vi "send_scan_data_to_AnalysisObj.vi"(0 "SessionID":string, 5 "plotname":string, 7 "magnet value in":dbl, 9 "value":dbl, 11 "error in (no error)":errorcluster) -> (15 "error out":errorcluster)   [LabVIEW 2017]
doc: "sendds the data to the AnalysisSession (SessionID) and stores them in the ScanDataArray"
uses:
  Classes/Analysis/Analysis.lvclass
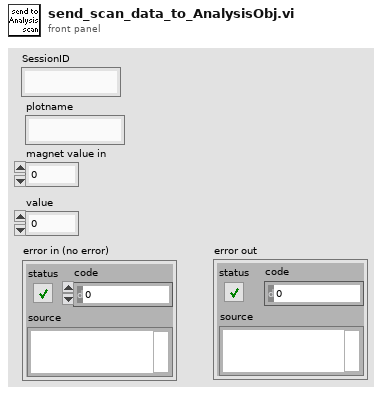
[diagram p1: front panel]
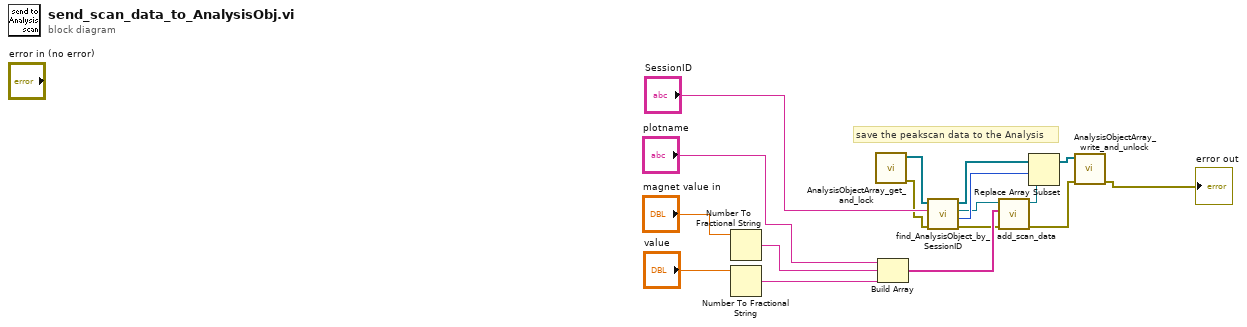
[diagram p0: block diagram]
diagram:
  # "save the peakscan data to the Analysis"
  n1 = Number To Fractional String(number="magnet value in") -> (F-format string=w14:string)  [unwired: 3 in]
  n2 = Number To Fractional String(number="value") -> (F-format string=w15:string)  [unwired: 3 in]
  n3 = call "AnalysisObjectArray_get_and_lock.vi"() -> ("error out"=w4:errorcluster, "AnalysisObjects"=w1:refnum<class "Analysis.lvclass">[])  [unwired: 10 in]
  n4 = Build Array("plotname", w14, w15) -> (w17:string[])
  n5 = call "find_AnalysisObject_by_SessionID.vi"("error in (no error)"=w4, "SessionID"="SessionID", "AnalysisObjects in"=w1) -> ("error out"=w3:errorcluster, "index of found"=w7:i32, "found AnalyisObject"=w2:refnum<class "Analysis.lvclass">, "AnalysisObjects out"=w5:refnum<class "Analysis.lvclass">[])  [unwired: 5 in]
  n6 = call-dynamic "add_scan_data.vi"("error in (no error)"=w3, "single scan data"=w17, "Analysis in"=w2) -> ("error out"=w9:errorcluster, "Analysis out"=w6:refnum<class "Analysis.lvclass">)  [unwired: 7 in]
  n7 = Replace Array Subset(array=w5, new element=w6, index=w7) -> (w8:refnum<class "Analysis.lvclass">[])
  n8 = call "AnalysisObjectArray_write_and_unlock.vi"("error in (no error)"=w9, "AnalysisObjects"=w8) -> ("error out"=→"error out":errorcluster)  [unwired: 9 in]
